vi "Nattify - Compute Bound on Grid.vi"(0 "grid size":i32, 5 "grid factor":i32, 7 "max location (not counting spacing and grid)":i32) -> (4 "computed bound on the grid":i32)   [LabVIEW 2020]
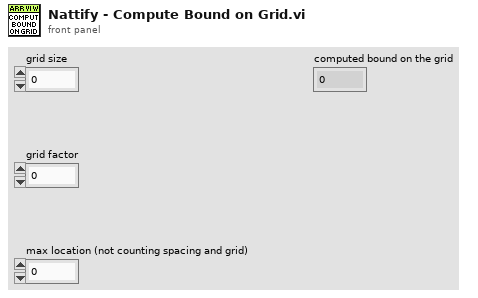
[diagram p1: front panel]
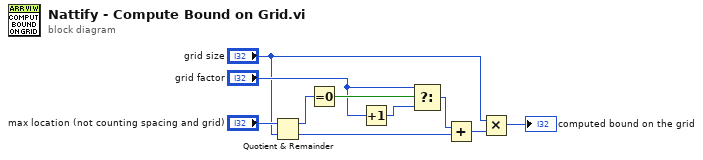
[diagram p0: block diagram]
diagram:
  n1 = Quotient & Remainder(x="max location (not counting spacing and grid)", y="grid size") -> (x-y*floor(x/y)=w2:i32, floor(x/y)=w1:i32)
  n2 = Equal To 0?(x=w2) -> (x = 0?=w9:bool)
  n3 = Increment(x="grid factor") -> (x+1=w8:i32)
  n4 = Select(t="grid factor", s=w9, f=w8) -> (s? t:f=w6:i32)
  n5 = Add(x=w6, y=w1) -> (x+y=w5:i32)
  n6 = Multiply(x="grid size", y=w5) -> (x*y=→"computed bound on the grid":i32)
